vi "test_btf_crest.vi"() -> ()   [LabVIEW 2014]
uses:
  common/crest/LabVIEW/LV14/libcommon-crest.lvlib
panel:
  out "timestamp":u64
  in  "stop":bool
  out "XY Graph":cluster{i32, dbl}[](graph)
  in  "cuname":string="BTF/QDC1"
  in  "chaoswanurl":string="192.168.150.91:8081"
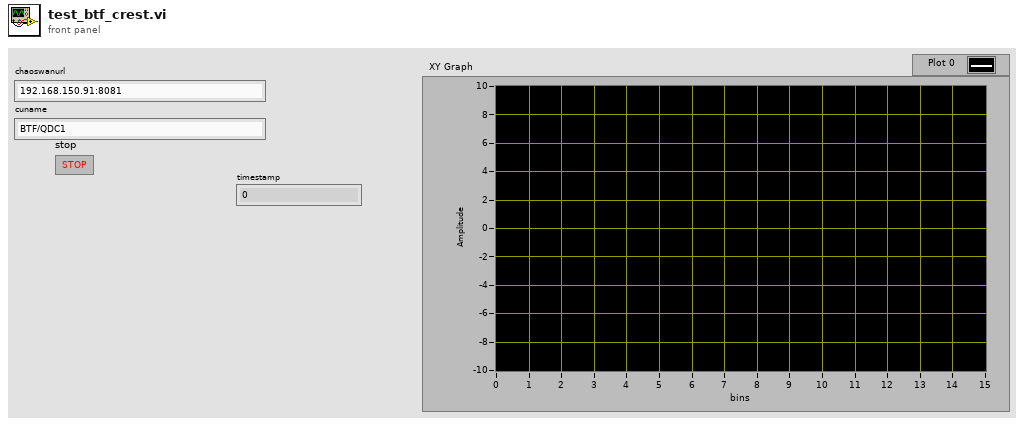
[diagram p1: front panel]
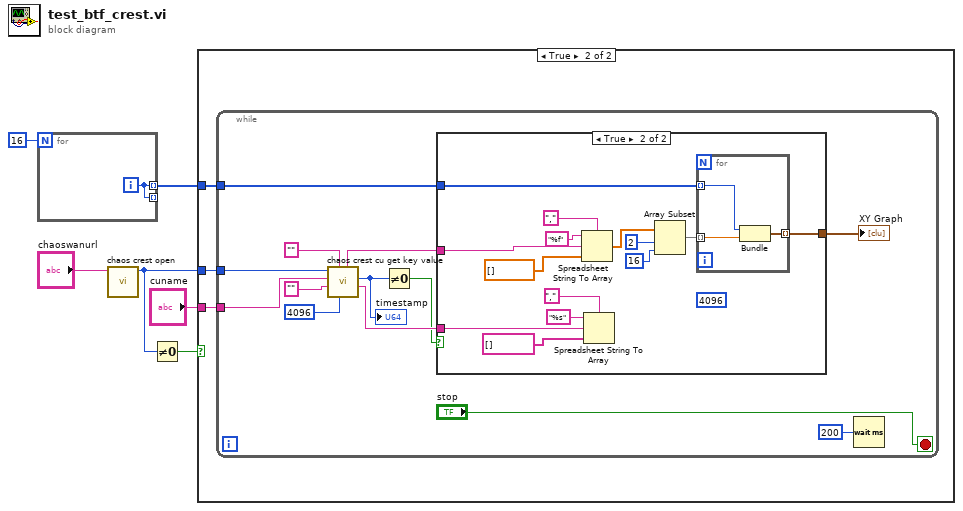
[diagram p0: block diagram]
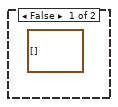
[diagram p2: hidden frame]
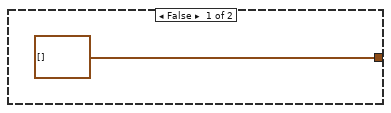
[diagram p3: hidden frame]
diagram:
  n1 = for {
    N: 16 -> [_]
    tunnel: [w7] -> _ mode=indexing
    tunnel: [w7] -> w1 mode=indexing
    i -> [w7]
  }
  n2 = call "chaos crest open.vi"("chaoswanurl"="chaoswanurl") -> ("handleConnection"=w4:u32)  [unwired: 10 in]
  n3 = Not Equal To 0?(x=w4) -> (x != 0?=w5:bool)
  n4 = case shown="True" w5 {
    tunnel: w4 -> [_ w10]
    tunnel: "cuname" -> [_ w9]
    tunnel: w1 -> [_ w8]
    frame False {
      (unwired) cluster{i32, dbl}[] []
    }
    frame True {
      n5 = while {
        tunnel: w10 -> [w23]
        tunnel: w9 -> [w22]
        tunnel: w8 -> [w16]
        stop <- "stop" stop-if-true
        n6 = call "chaos crest cu get key value.vi"("maxsize"=4096, "values"="", "keys"="" ("output"), "cuname"=w22, "handleConnection"=w23) -> ("keys out"=w17:string, "timestamp"=w15:u64, "values out"=w18:string)  [unwired: 3 in, 1 out]
        "timestamp" <- w15
        n7 = Not Equal To 0?(x=w15) -> (x != 0?=w14:bool)
        n8 = case shown="True" w14 {
          tunnel: w18 -> [_ w38]
          tunnel: w17 -> [_ w37]
          tunnel: w16 -> [_ w36]
          tunnel: [cluster{i32, dbl}[] [] w35] -> w11
          frame False {
          }
          frame True {
            (unwired) 4096 ("maxsize")
            n9 = Spreadsheet String To Array(delimiter (Tab)=",", format string="%f", spreadsheet string=w38, array type (2D Dbl)=dbl[] []) -> (array=w28:dbl[])
            n10 = Spreadsheet String To Array(delimiter (Tab)=",", format string="%s", spreadsheet string=w37, array type (2D Dbl)=string[] []) -> ()  [unwired: 1 out]
            n11 = Array Subset(array=w28, index=2, length=16) -> (w25:dbl[])
            n12 = for {
              tunnel: w25 -> [w41] mode=indexing
              tunnel: w36 -> [w40] mode=indexing
              tunnel: [w39] -> w35 mode=indexing
              n13 = Bundle(w40, w41) -> (w39:cluster{i32, dbl})  [unwired: 1 in]
            }
          }
        }
        "XY Graph" <- w11
        n14 = Wait (ms)(milliseconds to wait=u32 200) -> ()  [unwired: 1 out]
      }
    }
  }
